vi "4ptMovingAvg_v5.vi"(10 "Enable?":bool=TRUE, 11 "Raw input":fxp<+/-,26,5>) -> (3 "Avg. output":fxp<+/-,28,5>)   [LabVIEW 2020, in "MovingAvg.lvlib"]
doc: "4-point moving average of input signals (recursive)\n\nv2: In a SCTL to optimize resource usage"
uses:
  MovingAvg.lvlib
  <vilib>/Platform/TimedLoop/XDataNode/timing_clust.ctl
  <vilib>/Platform/TimedLoop/XDataNode/nitl_modes.ctl
  <vilib>/Platform/TimedLoop/XDataNode/wakeup.ctl
  <vilib>/rvi/Emulation/niFpgaSctlEmulationGetInTimedLoop.vi
  <vilib>/rvi/Emulation/niFpgaEmulationReportErrorSimple.vi
  <vilib>/rvi/Emulation/niFpgaGetClockAttributes.vi
  <vilib>/rvi/Emulation/niFpgaCriticalErrorInLSC.vi
  <vilib>/Platform/TimedLoop/XDataNode/XDataNode.xnode
  <vilib>/rvi/FXPMathLib/basic elements/FxpDiscreteDelay/XNode/nifxpmath_DiscreteDelay.xnode
  <vilib>/rvi/FXPMathLib/FxpSub/XNode/nifxpmath_Sub.xnode
  <vilib>/rvi/FXPMathLib/FxpAdd/XNode/nifxpmath_Add.xnode
  <vilib>/Platform/TimedLoop/XDataNode/XDNodeRunTimeDep.lvlib
  <vilib>/rvi/FXPMathLib/sim/FxpSim.dll
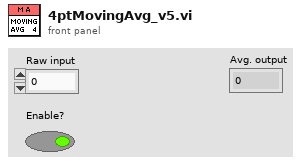
[diagram p1: front panel]
types:
  T1 = typedef "XDNodeRunTimeDep.lvlib/timing_clust.ctl" = cluster{"Expected End [f-1]":u64, "Actual End [f-1]":u64, "Finished Late? [f-1]":bool, "Expected End [i-1]":u64, "Actual End [i-1]":u64, "Finished Late? [i-1]":bool, "Expected Start [i]":u64, "Actual Start [i]":u64, "Expected Start [f]":u64, "Actual Start [f]":u64, "Source Name":string, "Structure Name":string, "Period":i64, "Deadline":i64, "Offset":i64, "Start":i64, "Priority":i32, "Timeout":i32, "Mode":T2, "Wakeup Reason":T3, "Error":errorcluster, "Source Type":string, "Secondary Source Type":string, "Global End Time":u64, "Global Start Time":u64, "Frame Duration":u64, "Iteration Duration":u64, "Assigned CPU":i32, "I/O Scan Engine Mode":u32}
  T2 = typedef "XDNodeRunTimeDep.lvlib/nitl_modes.ctl" = enum32{"No Change", "Process missed periods, maintain original phase", "Discard missed periods, maintain original phase", "Process missed periods, ignore original phase", "Discard missed periods, ignore original phase"}
  T3 = typedef "XDNodeRunTimeDep.lvlib/wakeup.ctl" = enum32{"Normal", "Aborted", "Asynchronous wakeup", "Timing source error", "Timed loop error", "Timeout"}
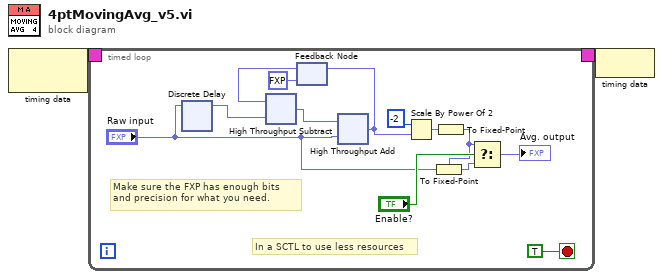
[diagram p0: block diagram]
diagram:
  n1 = node-c288() -> (w2:T1)  [unwired: 1 in]
  n2 = timed-loop {
    timing: w2 -> [_]
    timing-out: [_] -> w1
    stop <- TRUE stop-if-true
    # "In a SCTL to use less resources"
    # "Make sure the FXP has enough bits \nand precision for what you need."
    n3 = xnode ("Discrete Delay")("D"="Raw input") -> ("Q"=w10:fxp<+/-,26,5>)
    n4 = feedback #1(fxp<+/-,30,7> 0.0 ("x+y")) -> (w14:fxp<+/-,30,7>)
    n5 = xnode ("High Throughput Subtract")("x"=w14, "y"=w10) -> ("x-y"=w13:fxp<+/-,31,8>)
    n6 = xnode ("High Throughput Add")("x"=w13, "y"="Raw input") -> ("x+y"=w12:fxp<+/-,30,7>)
    n7 = feedback-in #1(w12) -> ()
    n8 = Scale By Power Of 2(n=i16 -2, x=w12) -> (x*2^n=w8:fxp<+/-,30,7>)
    n9 = To Fixed-Point(number=w8) -> (fixed-point=w3:fxp<+/-,28,5>)  [unwired: 1 in]
    n10 = To Fixed-Point(fixed-point type=w3, number="Raw input") -> (fixed-point=w7:fxp<+/-,28,5>)
    n11 = Select(t=w3, s="Enable?", f=w7) -> (s? t:f=→"Avg. output":fxp<+/-,28,5>)
  }
  n12 = node-c288(w1) -> ()
